vi "Variable length sanity check.vi"(10 "Number of miniscans":i32, 11 "VL X pixels":u16[](array[numeric])) -> ()   [LabVIEW 2020]
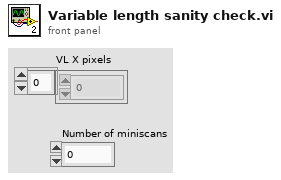
[diagram p1: front panel]
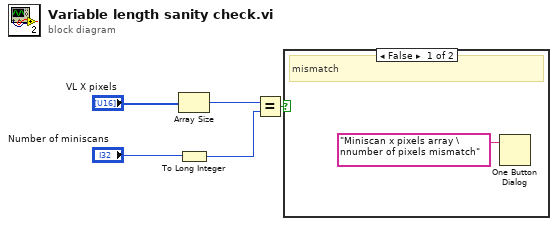
[diagram p0: block diagram]
diagram:
  n1 = Array Size(array="VL X pixels") -> (size(s)=w4:i32)
  n2 = To Long Integer(number="Number of miniscans") -> (32bit integer=w1:i32)
  n3 = Equal?(x=w4, y=w1) -> (x = y?=w3:bool)
  n4 = case shown="False" w3 {
    frame False {
      # "mismatch"
      n5 = One Button Dialog(message="Miniscan x pixels array \nnumber of pixels mismatch") -> ()  [unwired: 1 in, 1 out]
    }
    frame True {
      # "All OK"
    }
  }
